vi "Build Syslog Message.vi"(7 "Hostname":string, 8 "Severity Code":T2=enum."error", 9 "Facility Code":T1=enum."user", 10 "Message Content":string, 11 "Message Tag":string) -> (3 "Syslog Message":string)   [LabVIEW 2021, in "Event_Syslog.lvclass"]
uses:
  Event_Syslog.lvclass
  abs_EventLog/Support/Severity Code.ctl
  abs_EventLog/Support/Facility Code.ctl
  abs_EventLog/abs_EventLog.lvclass
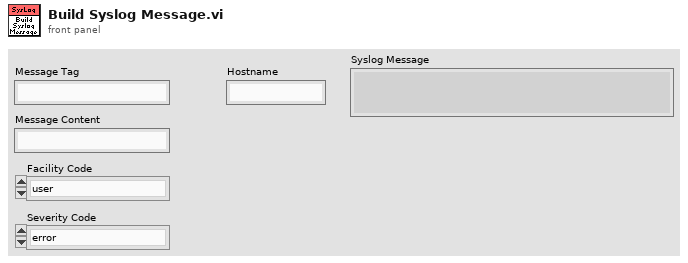
[diagram p1: front panel]
types:
  T1 = typedef "abs_EventLog.lvclass/Facility Code.ctl" = enum16{"kernel", "user", "mail", "system daemons", "security/authorization", "syslogd", "line printer", "network news", "uucp", "clock daemon", "security/authorization (alternate)", "FTP daemon", "NTP subsystem", "log audit", "log alert", "clock daemon (alternate)", "local use 0", "local use 1", "local use 2", "local use 3", "local use 4", "local use 5", "local use 6", "local use 7"}
  T2 = typedef "abs_EventLog.lvclass/Severity Code.ctl" = enum16{"emergency", "alert", "critical", "error", "warning", "notice", "info", "debug"}
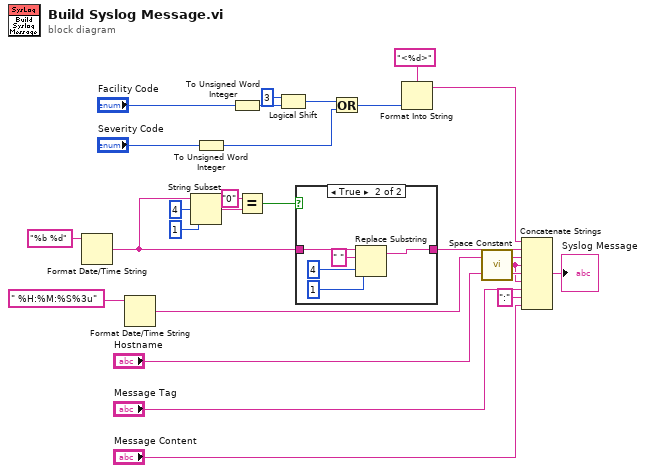
[diagram p0: block diagram]
diagram:
  n1 = Format Date/Time String(time format string (%c)="%b %d") -> (date/time string=w19:string)  [unwired: 2 in]
  n2 = Format Date/Time String(time format string (%c)=" %H:%M:%S%3u") -> (date/time string=w17:string)  [unwired: 2 in]
  n3 = String Subset(string=w19, offset (0)=4, length (rest)=1 ("length (rest)")) -> (substring=w22:string)
  n4 = To Unsigned Word Integer(number="Severity Code") -> (unsigned 16bit integer=w9:u16)
  n5 = To Unsigned Word Integer(number="Facility Code") -> (unsigned 16bit integer=w13:u16)
  n6 = Equal?(x="0", y=w22) -> (x = y?=w20:bool)
  n7 = Logical Shift(y=i16 3, x=w13) -> (x << y=w11:u16)
  n8 = case shown="True" w20 {
    tunnel: w19 -> [w26 w31]
    tunnel: [w26 w27] -> w18
    frame False {
    }
    frame True {
      n9 = Replace Substring(2:1 ("length (len. of substring)"), 3:4 ("offset (0)"), 4:" " ("substring (\"\")"), 5:w31) -> (1:w27:string)  [unwired: 1 out]
    }
  }
  n10 = Or(x=w11, y=w9) -> (x .or. y?=w8:u16)
  n11 = Format Into String(format string="<%d>", w8) -> (resulting string=w15:string)  [unwired: 2 in, 1 out]
  n12 = call <vilib>:"Space Constant.vi"() -> ("String"=w6:string)
  n13 = Concatenate Strings(w15, w18, w17, w6, "Hostname", w6, "Message Tag", ":" ("string"), "Message Content") -> (→"Syslog Message":string)
